vi "FindRectCenter.vi"(8 "Bottom":dbl, 9 "RIght":dbl, 10 "Top":dbl, 11 "Left":dbl) -> (0 "Y":dbl, 3 "X":dbl)   [LabVIEW 2016]
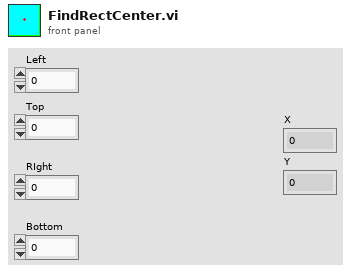
[diagram p1: front panel]
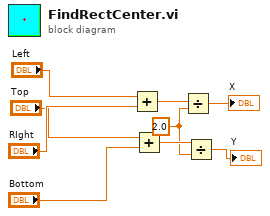
[diagram p0: block diagram]
diagram:
  w3 = 2.0 ("y")
  n1 = Add(x="Left", y="RIght") -> (x+y=w5:dbl)
  n2 = Add(x="Top", y="Bottom") -> (x+y=w4:dbl)
  n3 = Divide(x=w5, y=w3) -> (x/y=→"X":dbl)
  n4 = Divide(x=w4, y=w3) -> (x/y=→"Y":dbl)
